vi "time plot.vi"() -> ()   [LabVIEW 2024]
panel:
  out "Time plot 1/(1 + t)":cluster{dbl[], dbl[]}(graph)
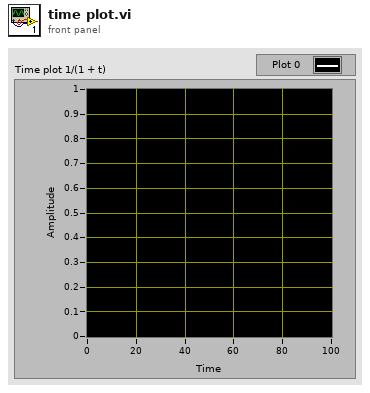
[diagram p1: front panel]
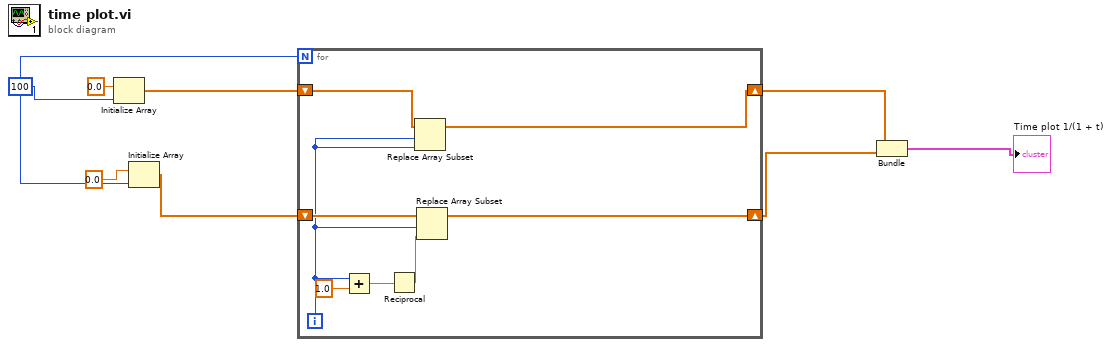
[diagram p0: block diagram]
diagram:
  w6 = 100
  n1 = Initialize Array(0.0 ("element"), w6) -> (w5:dbl[])
  n2 = Initialize Array(0.0 ("element"), w6) -> (w4:dbl[])
  n3 = for {
    N: w6 -> [_]
    shift-right: [w9] -> w3
    shift-left: w5 -> [w16]
    shift-right: [w10] -> w2
    shift-left: w4 -> [w15]
    i -> [w11]
    n4 = Add(x=w11, y=1.0) -> (x+y=w14:dbl)
    n5 = Reciprocal(x=w14) -> (1/x=w13:dbl)
    n6 = Replace Array Subset(array=w16, new element=w11, index=w11) -> (w9:dbl[])
    n7 = Replace Array Subset(array=w15, new element=w13, index=w11) -> (w10:dbl[])
  }
  n8 = Bundle(w3, w2) -> (→"Time plot 1/(1 + t)":cluster{dbl[], dbl[]})  [unwired: 1 in]
